vi "Volume 2012 NIVerified.vi"(6 "lpszWindowName":string, 8 "error in (no error)":errorcluster, 11 "Enum":enum16{"Mute", "Volume Up", "Volume Down"}(ring)) -> (0 "error out":errorcluster)   [LabVIEW 2012]
doc: "This example code first listens for button presses on the keyboard. If the correct key is pressed, the program executes a Windows API call through user32.dll to increase, decrease, or mute the volume"
uses:
  Windows/System32/user32.dll
panel:
  # "Overview:This example code first listens for button presses on the keyboard. If the correct key is \npressed, the program executes a Windows API call through user32.dll to increase, decrease, or mute the volume.\nRequirements:\nSoftware:\nLabVIEW 2012 SP1 or later\nInstructions:\n1.Ensure Volume 2012 NIVerified.vi is really running.\n2.Run the VI."
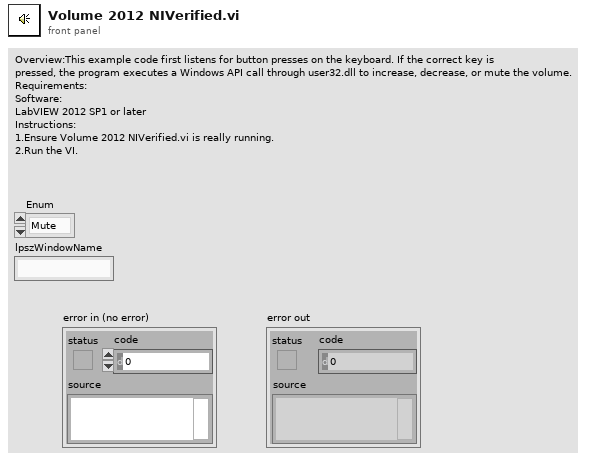
[diagram p1: front panel]
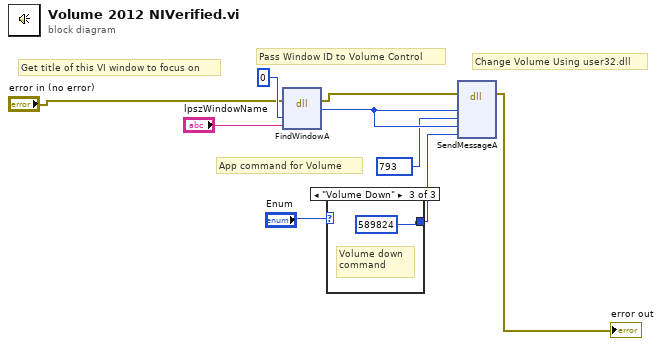
[diagram p0: block diagram]
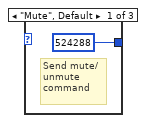
[diagram p2: hidden frame]
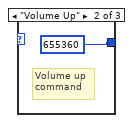
[diagram p3: hidden frame]
diagram:
  # "App command for Volume"
  # "Get title of this VI window to focus on"
  # "Pass Window ID to Volume Control"
  # "Change Volume Using user32.dll"
  n1 = dll-call lib="C:/Windows/System32/user32.dll" fn="FindWindowA"(error in="error in (no error)", "lpszClassName"=0, "lpszWindowName"="lpszWindowName") -> (error out=w4:errorcluster, "hWnd"=w8:u32)  [unwired: 4 in, 1 out]
  n2 = case shown="\"Volume Down\"" "Enum" {
    tunnel: [u32 524288 ("lParam") u32 655360 ("lParam") u32 589824 ("lParam")] -> w5
    frame "Mute", Default {
      # "Send mute/\nunmute \ncommand"
    }
    frame "Volume Up" {
      # "Volume up\ncommand"
    }
    frame "Volume Down" {
      # "Volume down\ncommand"
    }
  }
  n3 = dll-call lib="C:/Windows/System32/user32.dll" fn="SendMessageA"(error in=w4, "hWnd"=w8, "Msg"=u32 793, "wParam"=w8, "lParam"=w5) -> (error out=→"error out":errorcluster)  [unwired: 7 in, 1 out]
